vi "new.vi"(8 "error in":errorcluster, 11 "Websocket console plugin in":refnum<class "Websocket console plugin.lvclass">) -> (0 "error out":errorcluster, 3 "Websocket console plugin out":refnum<class "Websocket console plugin.lvclass">)   [LabVIEW 2016, in "Websocket console plugin.lvclass"]
uses:
  Websocket console plugin.lvclass
  Websocket console plugin.lvclass/Websocket console plugin.ctl
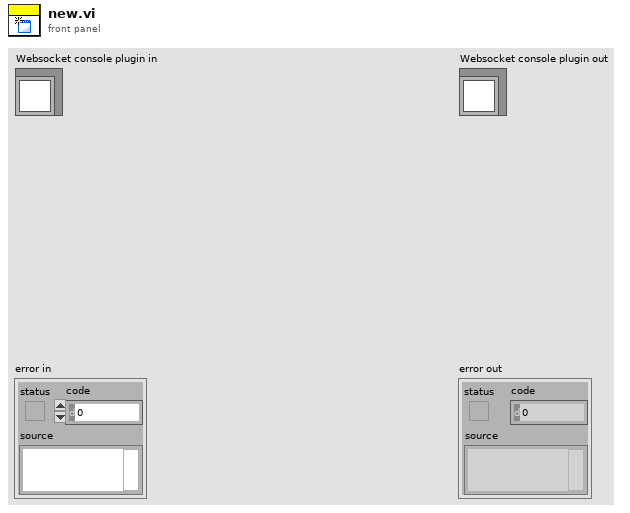
[diagram p1: front panel]
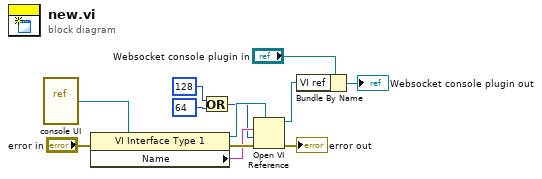
[diagram p0: block diagram]
diagram:
  n1 = vi-ref "console UI.vi"() -> (w1:refnum<vi>)
  n2 = property class="VI Interface Type 1"(reference=w1, error in="error in") -> (reference out=w9:refnum<vi>, error out=w11:errorcluster, "Name"=w10:string)
  n3 = Or(x=128 ("options"), y=64 ("options")) -> (x .or. y?=w8:i32)
  n4 = Open VI Reference(type specifier VI Refnum (for type only)=w9, vi path=w10, options=w8, error in (no error)=w11) -> (vi reference=w2:refnum<vi>, error out=→"error out":errorcluster)  [unwired: 2 in]
  n5 = Bundle By Name(cluster="Websocket console plugin in", "VI ref"=w2) -> (→"Websocket console plugin out":refnum<class "Websocket console plugin.lvclass">)
